vi "Requests.vi"(8 "error in (no error)":errorcluster, 9 "write enable":bool=TRUE, 11 "OHAUS in":refnum<class "OHAUS_Navigator.lvclass">) -> (0 "error out":errorcluster, 3 "OHAUS out":refnum<class "OHAUS_Navigator.lvclass">)   [LabVIEW 2021, in "OHAUS_Navigator.lvclass"]
uses:
  OHAUS_Navigator.lvclass
  Modbus_v121c/Network Interface/TCP Interface/TCP Shared Components/TCP Shared Components.lvlib
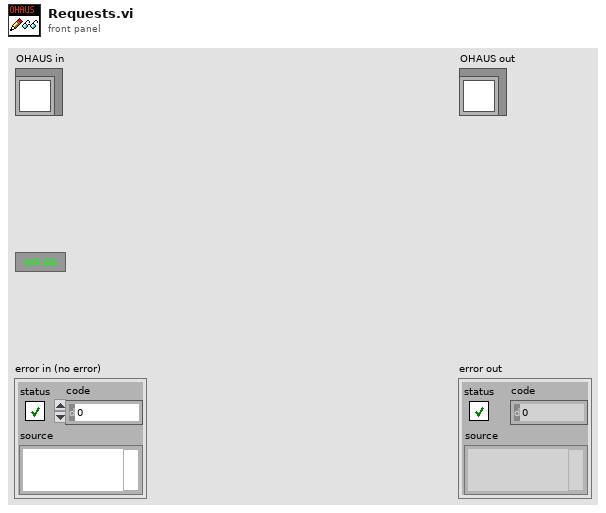
[diagram p1: front panel]
types:
  T1 = enum16{"Standard", "Buffered", "CRLF", "Immediate"}
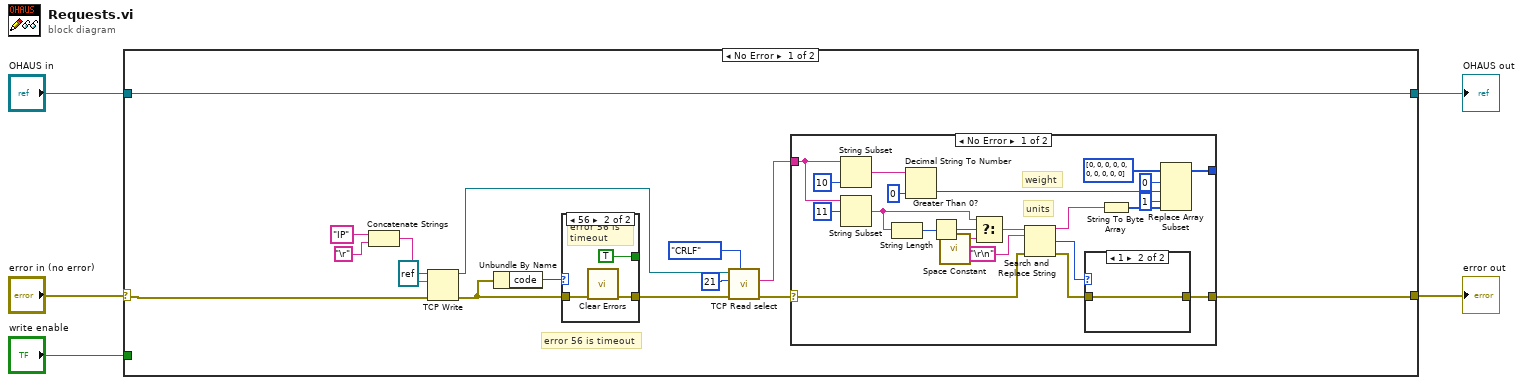
[diagram p0: block diagram]
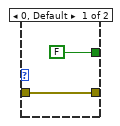
[diagram p2: hidden frame]
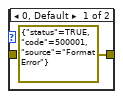
[diagram p3: hidden frame]
diagram:
  n1 = case shown="No Error" "error in (no error)" {
    selector: "error in (no error)" -> [w9 w52]
    tunnel: [w6 w52] -> w3
    tunnel: [w7 w51] -> w4
    tunnel: "OHAUS in" -> [w7 w51]
    tunnel: "write enable" -> [_ _]
    frame No Error {
      # "error 56 is timeout"
      n2 = Concatenate Strings("IP" ("Code"), "\r") -> (w16:string)
      n3 = TCP Write(connection ID=refnum<k5> refnum, data in=w16, error in (no error)=w9) -> (connection ID out=w12:refnum<k5>, error out=w18:errorcluster)  [unwired: 1 in, 1 out]
      n4 = Unbundle By Name(w18) -> ("code"=w17:i32)
      n5 = case shown="56" w17 {
        tunnel: w18 -> [w22 w24]
        tunnel: [w22 w23] -> w13
        tunnel: [FALSE TRUE] -> _
        frame 0, Default {
        }
        frame 56 {
          # "error 56 is timeout"
          n6 = call <vilib>:"Clear Errors.vi"("error in (no error)"=w24) -> ("error out"=w23:errorcluster)  [unwired: 5 in, 1 out]
        }
      }
      n7 = call "TCP Read select.vi"("mode (standard)"=T1."CRLF", "error in (no error)"=w13, "bytes to read"=21, "connection ID"=w12) -> ("error out"=w14:errorcluster, "data"=w11:string)  [unwired: 5 in, 1 out]
      n8 = case shown="No Error" w14 {
        selector: w14 -> [w29 w50]
        tunnel: w11 -> [w43 _]
        tunnel: [w27 w50] -> w6
        tunnel: [w34 _] -> _
        frame No Error {
          # "units"
          # "weight"
          n9 = String Subset(string=w43, length (rest)=10 ("length (rest)")) -> (substring=w45:string)  [unwired: 1 in]
          n10 = String Subset(string=w43, offset (0)=11 ("length (rest)")) -> (substring=w41:string)  [unwired: 1 in]
          n11 = String Length(string=w41) -> (length=w33:i32)
          n12 = Decimal String To Number(string=w45, default (0L)=0 ("default (0 I32)")) -> (number=w35:i32)  [unwired: 1 in, 1 out]
          n13 = Greater Than 0?(x=w33) -> (x > 0?=w42:bool)
          n14 = call <vilib>:"Space Constant.vi"() -> ("String"=w40:string)
          n15 = Select(t=w41, s=w42, f=w40) -> (s? t:f=w32:string)
          n16 = Search and Replace String(input string=w32, search string="\r\n", error in=w29) -> (result string=w31:string, number of replacements=w28:i32, error out=w26:errorcluster)  [unwired: 5 in, 1 out]
          n17 = case shown="1" w28 {
            tunnel: [errorcluster {"status"=TRUE, "code"=500001, "source"="Format Error"} ("error IO") w49] -> w27
            tunnel: w26 -> [_ w49]
            frame 0, Default {
            }
            frame 1 {
            }
          }
          n18 = String To Byte Array(string=w31) -> (unsigned byte array=w36:u8[])
          n19 = Replace Array Subset(array=u16[] [0, 0, 0, 0, 0, 0, 0, 0, 0, 0] ("Registers"), new element #1=w35, index #1=0 ("index"), new element #2=w36, index #2=1 ("index")) -> (w34:u16[])
        }
        frame Error {
        }
      }
    }
    frame Error {
    }
  }
  "error out" <- w3
  "OHAUS out" <- w4
